vi "conveyer mover.vi"() -> ()   [LabVIEW 2026]
panel:
  in  "stop":bool
  out "Slide":dbl(slide) scale=0.0..10.0
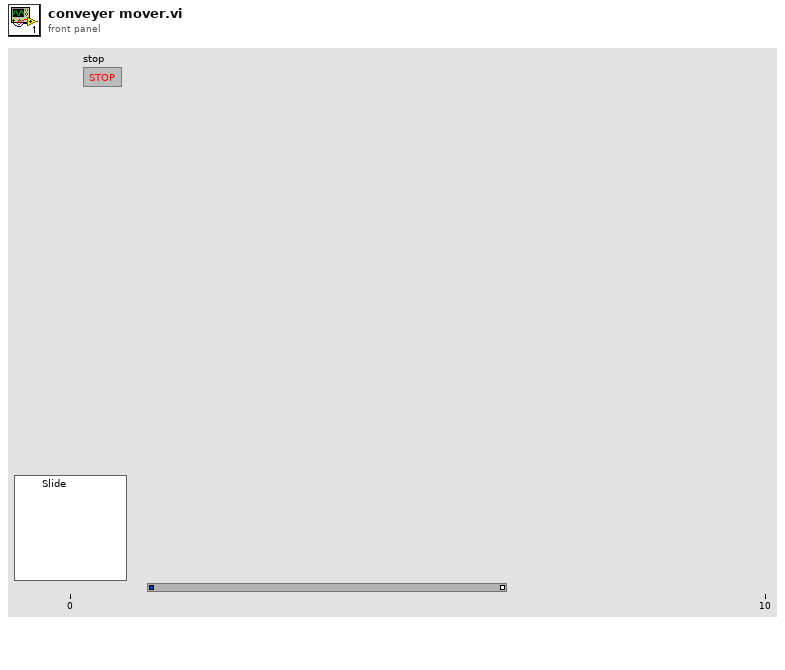
[diagram p1: front panel]
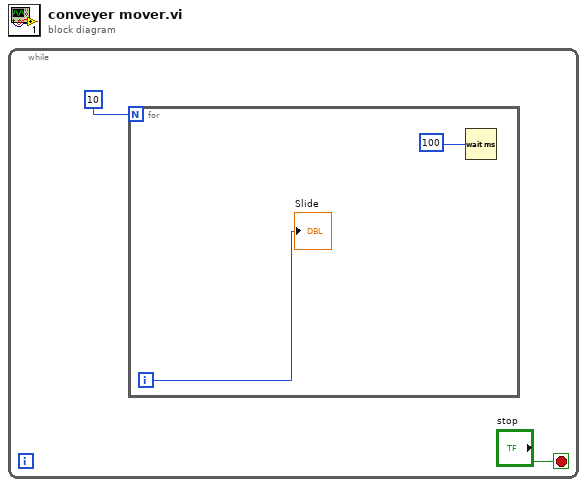
[diagram p0: block diagram]
diagram:
  n1 = while {
    stop <- "stop" stop-if-true
    n2 = for {
      N: 10 -> [_]
      i -> [w4]
      n3 = Wait (ms)(milliseconds to wait=u32 100) -> ()  [unwired: 1 out]
      "Slide" <- w4
    }
  }
